vi "get Motion.vi"(11 "Element in":refnum<class "Element.lvclass">) -> (3 "Motion":refnum<class "Motion.lvclass">)   [LabVIEW 2021, in "Element.lvclass"]
uses:
  Element.lvclass
  Motion/Motion.lvclass
  Element.lvclass/Element.ctl
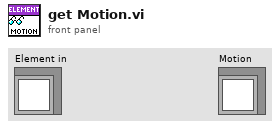
[diagram p1: front panel]
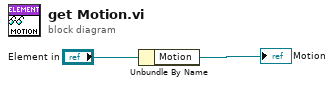
[diagram p0: block diagram]
diagram:
  n1 = Unbundle By Name("Element in") -> ("Motion"=→"Motion":refnum<class "Motion.lvclass">)
